vi "Emballage_BDD_lecture_CODE_GESTION_join_FiltreNoValve.vi"(8 "error in":errorcluster, 10 "ID_ARTICLE":i32, 11 "NOVALVE_FILTRE":string) -> (0 "error out":errorcluster, 1 "données Final":string[](array[string]), 2 "Colonne":string[](array[string])=["ID_ARTICLE_GPAO", "NOVALVE_FILTRE", "INDICE_PRODUIT", "AFFICHE_CODEBARRE_CLIENT", "MELANGE_LOT_POSSIBLE", "FAMILLE_VALVE", "REMARQUE"], 3 "tableauHeaders":string[][](array[string]))   [LabVIEW 2020]
uses:
  Modules/FS/60_FS_Controles/60_FS_SetGet.ctl
  <vilib>/addons/database/Connection.llb/DB Tools Open Connec (Path).vi
  <vilib>/addons/database/Connection.llb/Conn Execute.vi
  <vilib>/addons/database/Recordset.llb/Rec Fetch Recordset Data (R).vi
  <vilib>/addons/database/Recordset.llb/Rec Destroy - Connection.vi
  <vilib>/addons/database/NI_Database_API.lvlib
panel:
  out "CodeBarreFixeFin":string
  out "CodeBarreFixe":string
  out "Champs_GPAO 2":string
  out "Carac. Fin 2":string
  out "Carac. Fin":string
  out "Champs_GPAO":string
  out "données Table":string[](array[string])
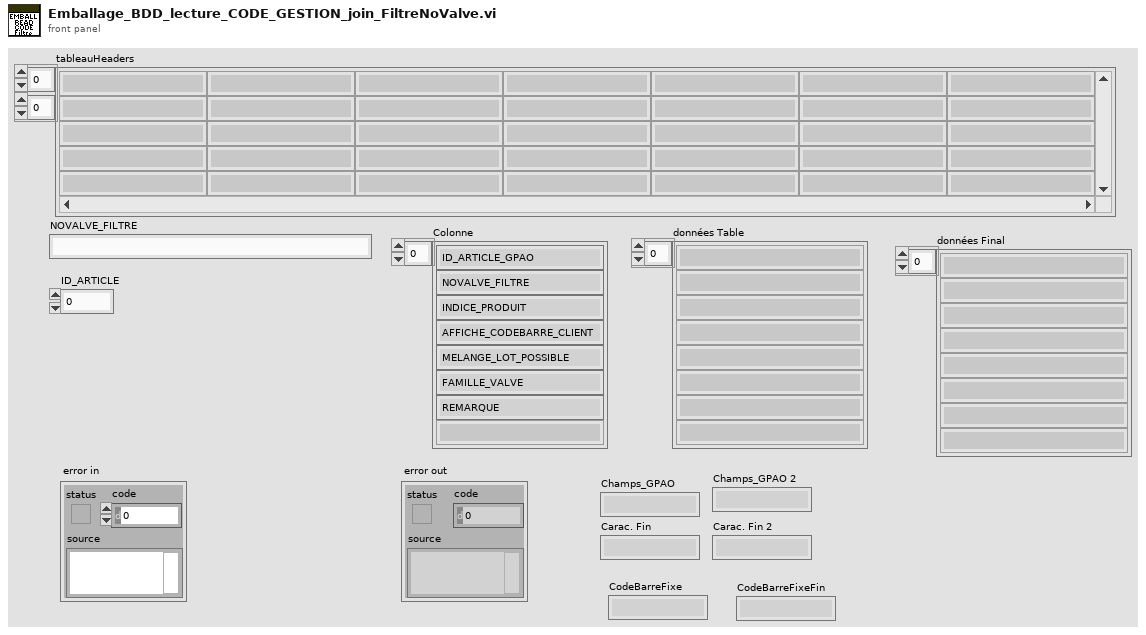
[diagram p1: front panel]
types:
  T1 = typedef "60_FS_SetGet.ctl" = enum16{"set", "get"}
  T2 = typedef "60_FS_CLT_Chemins.ctl" = cluster{"Racine_local":path, "Racine_reseau":path, "Racine_Support_Application":path, "Fichier_Journalisation":path, "Connexion_BDD_VSX":path, "Connexion_BDD_PLZ":path}
  T3 = typedef "NI_Database_API.lvlib/Conn ObjectReference.ctl" = refnum<k1>
  T4 = typedef "NI_Database_API.lvlib/Rec ObjectReference.ctl" = refnum<k1>
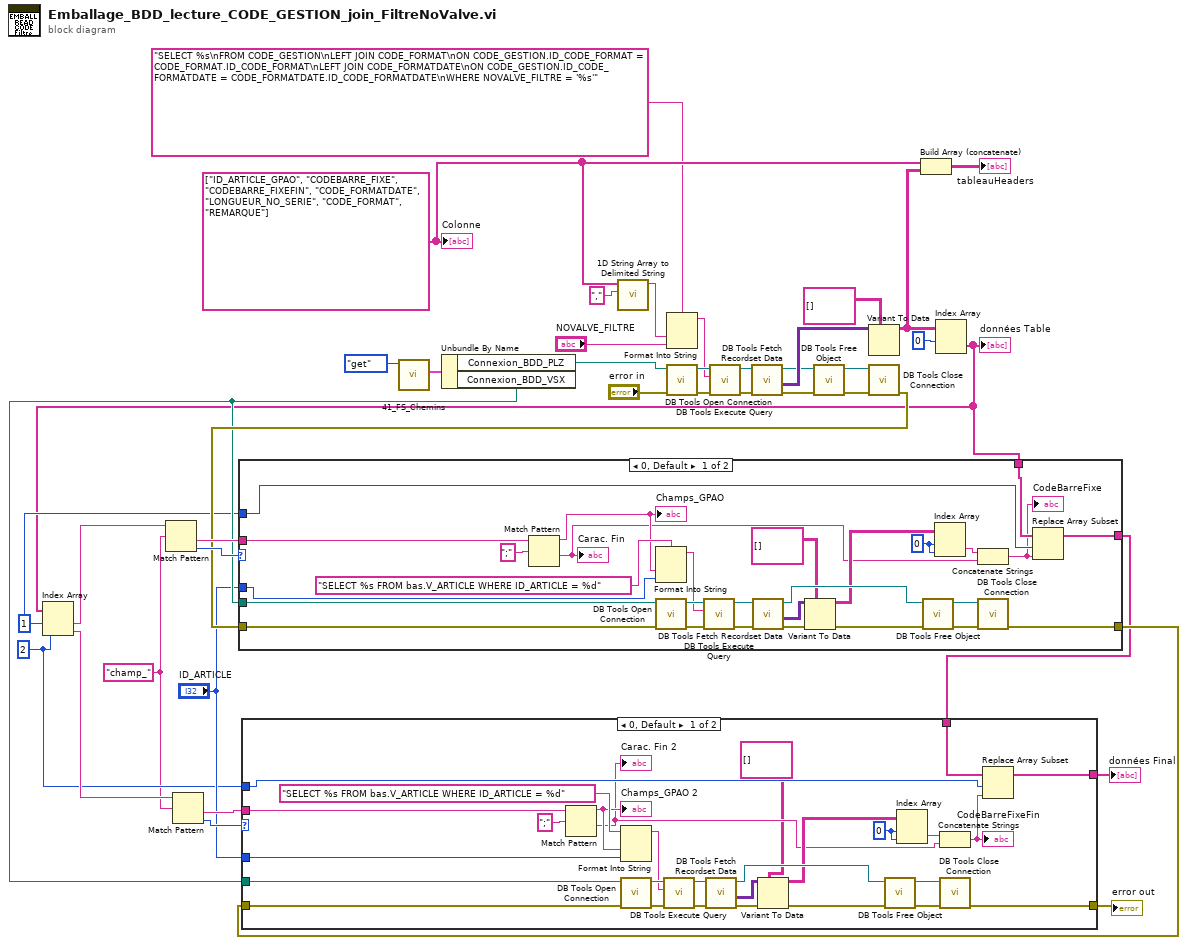
[diagram p0: block diagram]
diagram:
  w1 = "champ_" ("expression régulière")
  w3 = 2 ("index")
  w6 = 1 ("index")
  w24 = string[] ["ID_ARTICLE_GPAO", "CODEBARRE_FIXE", "CODEBARRE_FIXEFIN", "CODE_FORMATDATE", "LONGUEUR_NO_SERIE", "CODE_FORMAT", "REMARQUE"]
  n1 = call "41_FS_Chemins.vi"("SetGet"=60_FS_SetGet."get") -> ("CLT_Chemins_out"=w26:T2)  [unwired: 9 in, 1 out]
  n2 = Unbundle By Name(w26) -> ("Connexion_BDD_PLZ"=w25:path, "Connexion_BDD_VSX"=w10:path)
  n3 = call <vilib>:"1D String Array to Delimited String.vi"("delimiter"=",", "string array"=w24) -> ("delimited string"=w20:string)  [unwired: 9 in]
  n4 = Format Into String(format string="SELECT %s\nFROM CODE_GESTION\nLEFT JOIN CODE_FORMAT\nON CODE_GESTION.ID_CODE_FORMAT = CODE_FORMAT.ID_CODE_FORMAT\nLEFT JOIN CODE_FORMATDATE\nON CODE_GESTION.ID_CODE_FORMATDATE = CODE_FORMATDATE.ID_CODE_FORMATDATE\nWHERE NOVALVE_FILTRE = '%s'" ("SQL query"), w20, "NOVALVE_FILTRE") -> (resulting string=w22:string)  [unwired: 2 in, 1 out]
  n5 = call-poly <vilib>:"DB Tools Open Connection.vi"("error in (no error)"="error in", "connection information"=w25) -> ("error out"=w30:errorcluster, "connection reference"=w31:T3)  [unwired: 6 in]
  n6 = call-poly <vilib>:"DB Tools Execute Query.vi"("error in (no error)"=w30, "SQL query"=w22, "connection reference"=w31) -> ("error out"=w39:errorcluster, "recordset reference"=w32:T4)  [unwired: 5 in]
  n7 = call-poly <vilib>:"DB Tools Fetch Recordset Data.vi"("error in (no error)"=w39, "recordset reference"=w32) -> ("error out"=w35:errorcluster, "recordset data"=w38:variant[][], "recordset reference out"=w36:T4)  [unwired: 3 in]
  n8 = call-poly <vilib>:"DB Tools Free Object.vi"("error in (no error)"=w35, "recordset reference"=w36) -> ("error out"=w34:errorcluster, "connection reference"=w33:T3)  [unwired: 8 in]
  n9 = Variant To Data(type=string[][] [] ("Liste des champs à lire 2"), Variant=w38) -> (data=w29:string[][])  [unwired: 1 in, 1 out]
  n10 = call <vilib>:"DB Tools Close Connection.vi"("error in (no error)"=w34, "connection reference"=w33) -> ("error out"=w11:errorcluster)  [unwired: 5 in]
  n11 = Build Array (concatenate)(w24, w29) -> (→"tableauHeaders":string[][])
  n12 = Index Array(array=w29, index (row)=0 ("indice (ligne)")) -> (element=w5:string[])  [unwired: 1 in]
  "données Table" <- w5
  n13 = Index Array(array=w5, index #1=w6, index #2=w3) -> (element #1=w17:string, element #2=w15:string)
  n14 = Match Pattern(string=w17, regular expression=w1) -> (after substring=w13:string, offset past match=w16:i32)  [unwired: 1 in, 2 out]
  n15 = Match Pattern(string=w15, regular expression=w1) -> (after substring=w12:string, offset past match=w14:i32)  [unwired: 1 in, 2 out]
  n16 = case shown="0, Default" w16 {
    tunnel: w13 -> [w67 _]
    tunnel: w11 -> [w58 w70]
    tunnel: w10 -> [w57 _]
    tunnel: [w56 w70] -> w9
    tunnel: "ID_ARTICLE" -> [w53 _]
    tunnel: w5 -> [w45 w69]
    tunnel: w6 -> [w44 _]
    tunnel: [w42 w69] -> w4
    frame 0, Default {
      w48 = 0 ("index (row)")
      n17 = Match Pattern(string=w67, regular expression=";" ("expression régulière")) -> (before substring=w54:string, after substring=w46:string)  [unwired: 1 in, 2 out]
      "Champs_GPAO" <- w54
      "Carac. Fin" <- w46
      n18 = Format Into String(format string="SELECT %s FROM bas.V_ARTICLE WHERE ID_ARTICLE = %d" ("Requète"), w54, w53) -> (resulting string=w52:string)  [unwired: 2 in, 1 out]
      n19 = call-poly <vilib>:"DB Tools Open Connection.vi"("error in (no error)"=w58, "connection information"=w57) -> ("error out"=w64:errorcluster, "connection reference"=w63:T3)  [unwired: 6 in]
      n20 = call-poly <vilib>:"DB Tools Execute Query.vi"("error in (no error)"=w64, "SQL query"=w52, "connection reference"=w63) -> ("error out"=w59:errorcluster, "recordset reference"=w60:T4)  [unwired: 5 in]
      n21 = call-poly <vilib>:"DB Tools Fetch Recordset Data.vi"("error in (no error)"=w59, "recordset reference"=w60) -> ("error out"=w62:errorcluster, "recordset data"=w61:variant[][], "recordset reference out"=w51:T4)  [unwired: 3 in]
      n22 = Variant To Data(error in=w62, type=string[][] [] ("Liste des champs à lire 2"), Variant=w61) -> (data=w49:string[][], error out=w65:errorcluster)
      n23 = call-poly <vilib>:"DB Tools Free Object.vi"("error in (no error)"=w65, "recordset reference"=w51) -> ("error out"=w66:errorcluster, "connection reference"=w50:T3)  [unwired: 8 in]
      n24 = Index Array(array=w49, index (row)=w48, index (col)=w48) -> (element=w47:string)
      n25 = Concatenate Strings(w47, w46) -> (w43:string)
      "CodeBarreFixe" <- w43
      n26 = call <vilib>:"DB Tools Close Connection.vi"("error in (no error)"=w66, "connection reference"=w50) -> ("error out"=w56:errorcluster)  [unwired: 5 in]
      n27 = Replace Array Subset(array=w45, new element=w43, index=w44) -> (w42:string[])
    }
    frame -1 {
    }
  }
  n28 = case shown="0, Default" w14 {
    tunnel: w12 -> [w97 _]
    tunnel: w10 -> [w88 _]
    tunnel: w9 -> [w87 w100]
    tunnel: [w86 w100] -> w8
    tunnel: "ID_ARTICLE" -> [w83 _]
    tunnel: w4 -> [w76 w99]
    tunnel: w3 -> [w75 _]
    tunnel: [w73 w99] -> w2
    frame 0, Default {
      w77 = 0 ("index (row)")
      n29 = Match Pattern(string=w97, regular expression=";" ("expression régulière")) -> (before substring=w84:string, after substring=w72:string)  [unwired: 1 in, 2 out]
      "Champs_GPAO 2" <- w84
      "Carac. Fin 2" <- w72
      n30 = Format Into String(initial string="SELECT %s FROM bas.V_ARTICLE WHERE ID_ARTICLE = %d" ("Requète"), w84, w83) -> (resulting string=w82:string)  [unwired: 2 in, 1 out]
      n31 = call-poly <vilib>:"DB Tools Open Connection.vi"("error in (no error)"=w87, "connection information"=w88) -> ("error out"=w91:errorcluster, "connection reference"=w92:T3)  [unwired: 6 in]
      n32 = call-poly <vilib>:"DB Tools Execute Query.vi"("error in (no error)"=w91, "SQL query"=w82, "connection reference"=w92) -> ("error out"=w96:errorcluster, "recordset reference"=w95:T4)  [unwired: 5 in]
      n33 = call-poly <vilib>:"DB Tools Fetch Recordset Data.vi"("error in (no error)"=w96, "recordset reference"=w95) -> ("error out"=w93:errorcluster, "recordset data"=w94:variant[][], "recordset reference out"=w81:T4)  [unwired: 3 in]
      n34 = Variant To Data(error in=w93, type=string[][] [] ("Liste des champs à lire 2"), Variant=w94) -> (data=w78:string[][], error out=w90:errorcluster)
      n35 = call-poly <vilib>:"DB Tools Free Object.vi"("error in (no error)"=w90, "recordset reference"=w81) -> ("error out"=w89:errorcluster, "connection reference"=w80:T3)  [unwired: 8 in]
      n36 = Index Array(array=w78, index (row)=w77, index (col)=w77) -> (element=w79:string)
      n37 = Concatenate Strings(w79, w72) -> (w74:string)
      "CodeBarreFixeFin" <- w74
      n38 = call <vilib>:"DB Tools Close Connection.vi"("error in (no error)"=w89, "connection reference"=w80) -> ("error out"=w86:errorcluster)  [unwired: 5 in]
      n39 = Replace Array Subset(array=w76, new element=w74, index=w75) -> (w73:string[])
    }
    frame -1 {
    }
  }
  "error out" <- w8
  "données Final" <- w2
  "Colonne" <- w24
